vi "Scope Tester.vi"() -> ()   [LabVIEW 2024]
uses:
  Logger/Logger.lvclass
  Log Levels.ctl
  Logging.lvlib
  Scope Tester Class.lvclass
  Scope Tester Library.lvlib
  Filters/Scopes/Basic/Basic.lvclass
  Filters/Scopes/Basic/New (Element).vi
  Logger/Internal Log Levels.ctl
  Log Record.ctl
panel:
  out "error out":errorcluster
  out "fail info":T3 {"Log Record"."timestamp" format="%<%x %.3X>T"}
  # "Locals"
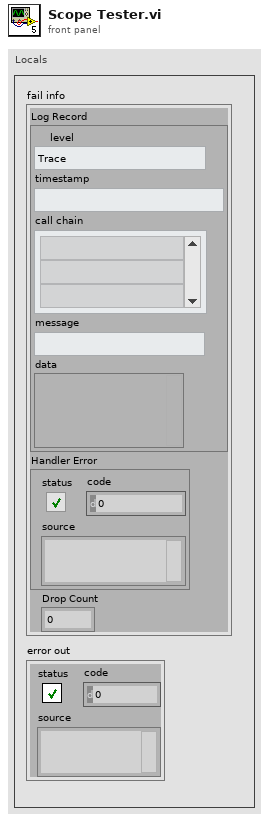
[diagram p1: front panel]
types:
  T1 = typedef "Logging.lvlib/Log Record.ctl" = cluster{"level":T2, "timestamp":timestamp, "call chain":string[], "message":string, "data":variant}
  T2 = typedef "Logging.lvlib/Internal Log Levels.ctl" = enum16{"Trace", "Debug", "Info", "Warning", "Error", "Critical", "Internal"}
  T3 = cluster{"Log Record":T1, "Handler Error":errorcluster, "Drop Count":u32}
  T4 = typedef "Logging.lvlib/Log Levels.ctl" = enum16{"Trace", "Debug", "Info", "Warning", "Error", "Critical"}
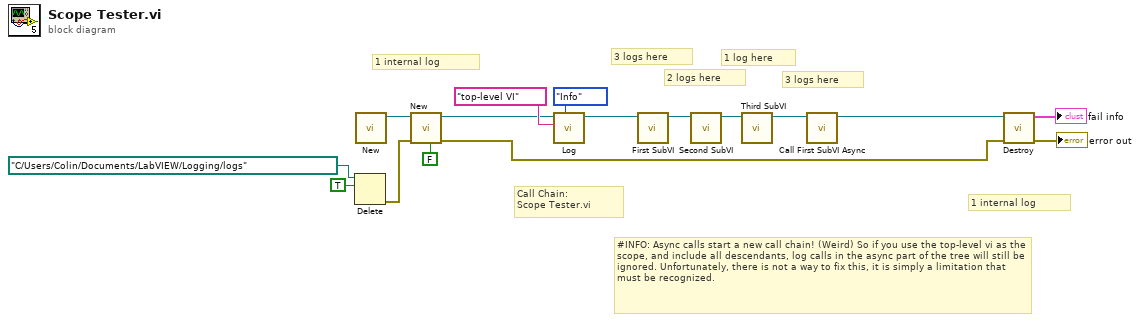
[diagram p0: block diagram]
diagram:
  # "#INFO: Async calls start a new call chain! (Weird) So if you use the top-level vi as the scope, and include all descendants, log calls in the async part of the tree will still be ignored. Unfortunately, there is not a way to fix this, it is simply a limitation that must be recognized."
  # "3 logs here"
  # "1 log here"
  # "2 logs here"
  # "1 internal log"
  # "3 logs here"
  # "Call Chain:\nScope Tester.vi"
  # "1 internal log"
  n1 = Delete(path (use dialog)=path "C:/Users/Colin/Documents/LabVIEW/Logging/logs", entire hierarchy (F)=TRUE) -> (error out=w5:errorcluster)  [unwired: 3 in, 2 out]
  n2 = call-poly "New.vi"() -> ("basic scope"=w16:refnum<class "Basic.lvclass">)  [unwired: 11 in]
  n3 = call "New.vi"("dialog on failure? (T)"=FALSE, "error in (no error)"=w5, "logger scope (all)"=w16) -> ("error out"=w10:errorcluster, "logger"=w14:refnum<class "Logger.lvclass">)  [unwired: 7 in]
  n4 = call "Log.vi"("log level"=Log_Levels."Info" ("level"), "message"="top-level VI", "logger in"=w14) -> ("logger out"=w12:refnum<class "Logger.lvclass">)  [unwired: 8 in]
  n5 = call "First SubVI.vi"("logger in"=w12) -> ("logger out"=w4:refnum<class "Logger.lvclass">)  [unwired: 10 in]
  n6 = call "Second SubVI.vi"("logger in"=w4) -> ("logger out"=w3:refnum<class "Logger.lvclass">)  [unwired: 10 in]
  n7 = call "Third SubVI.vi"("logger in"=w3) -> ("logger out"=w2:refnum<class "Logger.lvclass">)  [unwired: 10 in]
  n8 = call "Call First SubVI Async.vi"("logger in"=w2) -> ("logger out"=w1:refnum<class "Logger.lvclass">)  [unwired: 10 in]
  n9 = call "Destroy.vi"("error in (no error)"=w10, "logger in"=w1) -> ("error out"=→"error out":errorcluster, "fail info"=→"fail info":T3)  [unwired: 8 in]
